vi "example_GMotionComplete.vi"() -> ()   [LabVIEW 2020]
uses:
  resources/gclibo32/gclibo32.lvlib
  resources/gclib32/gclib32.lvlib
panel:
  out "Reference Position":string="\r\n:"
  in  "Command 2":string="MG_RPA"
  out "Error Out":errorcluster
  in  "IP Address":string="192.168.1.77"
  in  "Command":string="SHA;PAA=4000;BGA"
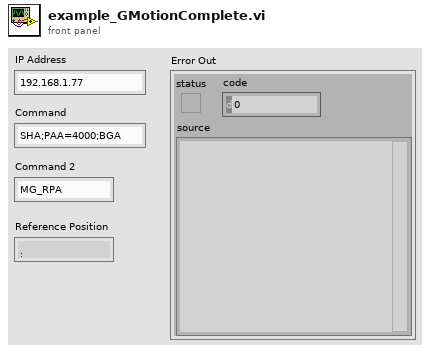
[diagram p1: front panel]
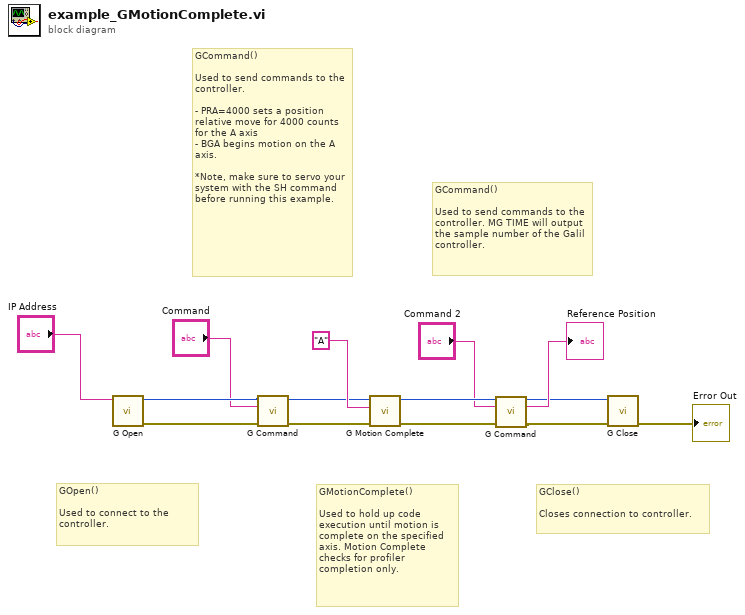
[diagram p0: block diagram]
diagram:
  # "GCommand()\n\nUsed to send commands to the controller. MG TIME will output the sample number of the Galil controller."
  # "GMotionComplete()\n\nUsed to hold up code execution until motion is complete on the specified axis. Motion Complete checks for profiler completion only."
  # "GClose()\n\nCloses connection to controller."
  # "GCommand()\n\nUsed to send commands to the controller. \n\n- PRA=4000 sets a position relative move for 4000 counts for the A axis\n- BGA begins motion on the A axis.\n\n*Note, make sure to servo your system with the SH command before running this example."
  # "GOpen()\n\nUsed to connect to the controller."
  n1 = call "G Open.vi"("address"="IP Address") -> ("error out"=w9:errorcluster, "g out"=w11:u32)  [unwired: 8 in]
  n2 = call "G Command.vi"("g"=w11, "command"="Command", "error in (no error)"=w9) -> ("g out"=w7:u32, "error out"=w8:errorcluster)  [unwired: 10 in, 1 out]
  n3 = call "G Motion Complete.vi"("error in (no error)"=w8, "axes"="A", "g"=w7) -> ("error out"=w5:errorcluster, "g out"=w6:u32)  [unwired: 7 in]
  n4 = call "G Command.vi"("g"=w6, "command"="Command 2", "error in (no error)"=w5) -> ("g out"=w2:u32, "buffer out"=→"Reference Position":string, "error out"=w1:errorcluster)  [unwired: 10 in]
  n5 = call "G Close.vi"("error in (no error)"=w1, "g"=w2) -> ("error out"=→"Error Out":errorcluster)  [unwired: 9 in]
